vi "Init Runtime.vi"(8 "error in (no error)":errorcluster, 10 "data allocations":T1, 11 "Conditional Jump Step Config in":refnum<class "Conditional Jump Step Config.lvclass">) -> (0 "error out":errorcluster, 2 "Skip":bool, 3 "Conditional Jump Step Config out":refnum<class "Conditional Jump Step Config.lvclass">)   [LabVIEW 2015, in "Conditional Jump Step Config.lvclass"]
uses:
  Conditional Jump Step Config.lvclass
  <vilib>/NI/Tag Bus Module Framework/channel/data tables.ctl
  <vilib>/NI/Tag Bus/dictionary/data dictionary.lvclass
  <vilib>/NI/Tag Bus/dictionary table pair.ctl
  <vilib>/NI/Tag Bus/table/data table.ctl
  Conditional Jump Step/Conditional Jump Step.lvclass
  <vilib>/NI/Tag Bus/tag/tag descriptor.lvclass/tag descriptor.ctl
  <vilib>/NI/Tag Bus/tag/read tag name.vi
  <vilib>/NI/Tag Bus/tag/read data type.vi
  <vilib>/NI/Tag Bus/dictionary/locate tag.vi
  <vilib>/NI/Tag Bus Module Framework/channel/TBM channel.lvclass
  <vilib>/NI/Tag Bus/table/data table.lvlib
  <vilib>/NI/Tag Bus/tag bus.lvlib
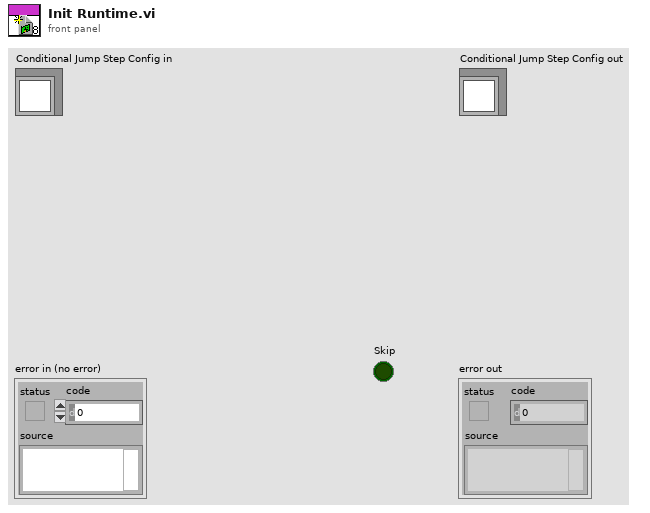
[diagram p1: front panel]
types:
  T1 = typedef "TBM channel.lvclass/data tables.ctl" = cluster{"input data":T2, "processing parameter":T2, "processing result":T2, "output data":T2}
  T2 = typedef "tag bus.lvlib/dictionary table pair.ctl" = cluster{"data dictionary":refnum<class "data dictionary.lvclass">, "data table":T3}
  T3 = typedef "tag bus.lvlib/data table.lvlib/data table.ctl" = cluster{"Double":dbl[], "Single":sgl[], "I64":i64[], "I32":i32[], "I16":i16[], "I8":i8[], "U64":u64[], "U32":u32[], "U16":u16[], "U8":u8[], "Boolean":bool[], "String":string[], "Array of Double":cluster{"DBL Array":dbl[]}[], "Array of Single":cluster{"SGL Array":sgl[]}[], "Array of I64":cluster{"I64 Array":i64[]}[], "Array of I32":cluster{"I32 Array":i32[]}[], "Array of I16":cluster{"I16 Array":i16[]}[], "Array of I8":cluster{"I8 Array":i8[]}[], "Array of U64":cluster{"U64 Array":u64[]}[], "Array of U32":cluster{"U32 Array":u32[]}[], "Array of U16":cluster{"U16 Array":u16[]}[], "Array of U8":cluster{"U8 Array":u8[]}[], "Array of Boolean":cluster{"Boolean Array":bool[]}[], "Array of String":cluster{"String Array":string[]}[]}
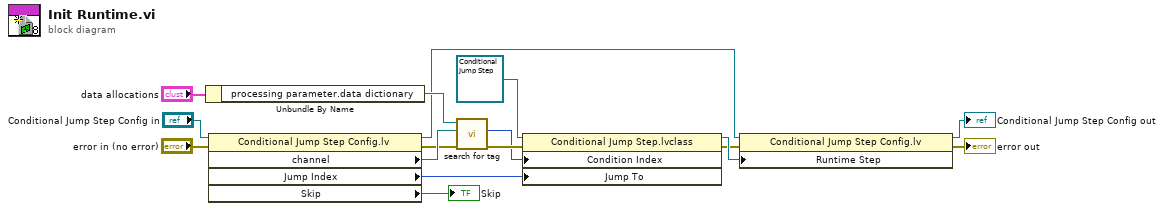
[diagram p0: block diagram]
diagram:
  n1 = Unbundle By Name("data allocations") -> ("processing parameter.data dictionary"=w14:refnum<class "data dictionary.lvclass">)
  n2 = property class="Conditional Jump Step Config.lv"(reference="Conditional Jump Step Config in", error in="error in (no error)") -> (reference out=w9:refnum<class "Conditional Jump Step Config.lvclass">, error out=w4:errorcluster, "channel"=w13:refnum<class "TBM channel.lvclass">, "Jump Index"=w1:i32, "Skip"=→"Skip":bool)
  n3 = call <vilib>:"search for tag.vi"("error in"=w4, "system tag"=w13, "data dictionary in"=w14) -> ("error out"=w3:errorcluster, "index"=w2:i32)  [unwired: 6 in, 1 out]
  n4 = property class="Conditional Jump Step.lvclass"(reference=refnum<class "Conditional Jump Step.lvclass"> refnum ("Conditional Jump Step.lvclass"), error in=w3, "Condition Index"=w2, "Jump To"=w1) -> (reference out=w12:refnum<class "Conditional Jump Step.lvclass">, error out=w11:errorcluster)
  n5 = property class="Conditional Jump Step Config.lv"(reference=w9, error in=w11, "Runtime Step"=w12) -> (reference out=→"Conditional Jump Step Config out":refnum<class "Conditional Jump Step Config.lvclass">, error out=→"error out":errorcluster)
